vi "Give_Name_Cluster(Img_Setting)-1.vi"() -> (1 "Histogram Settings":T2, 2 "Image Settings":T1)   [LabVIEW 2013]
panel:
  in  "Expanding Factor":u16=700
  in  "Inverse #2":bool=TRUE
  in  "Inverse #1":bool=TRUE
  in  "Shift #2":u16
  in  "Shift #1":u16
  in  "Sigma #2":dbl=2.5
  in  "Dim #2":u8=15
  in  "Sigma #1":dbl=2.5
  in  "Dim #1":u8=15
  in  "Operator #2":T3(ring)
  in  "Intensity #2":sgl format="%.2f"
  in  "Operator #1":T3(ring)
  in  "Intensity #1":sgl format="%.2f"
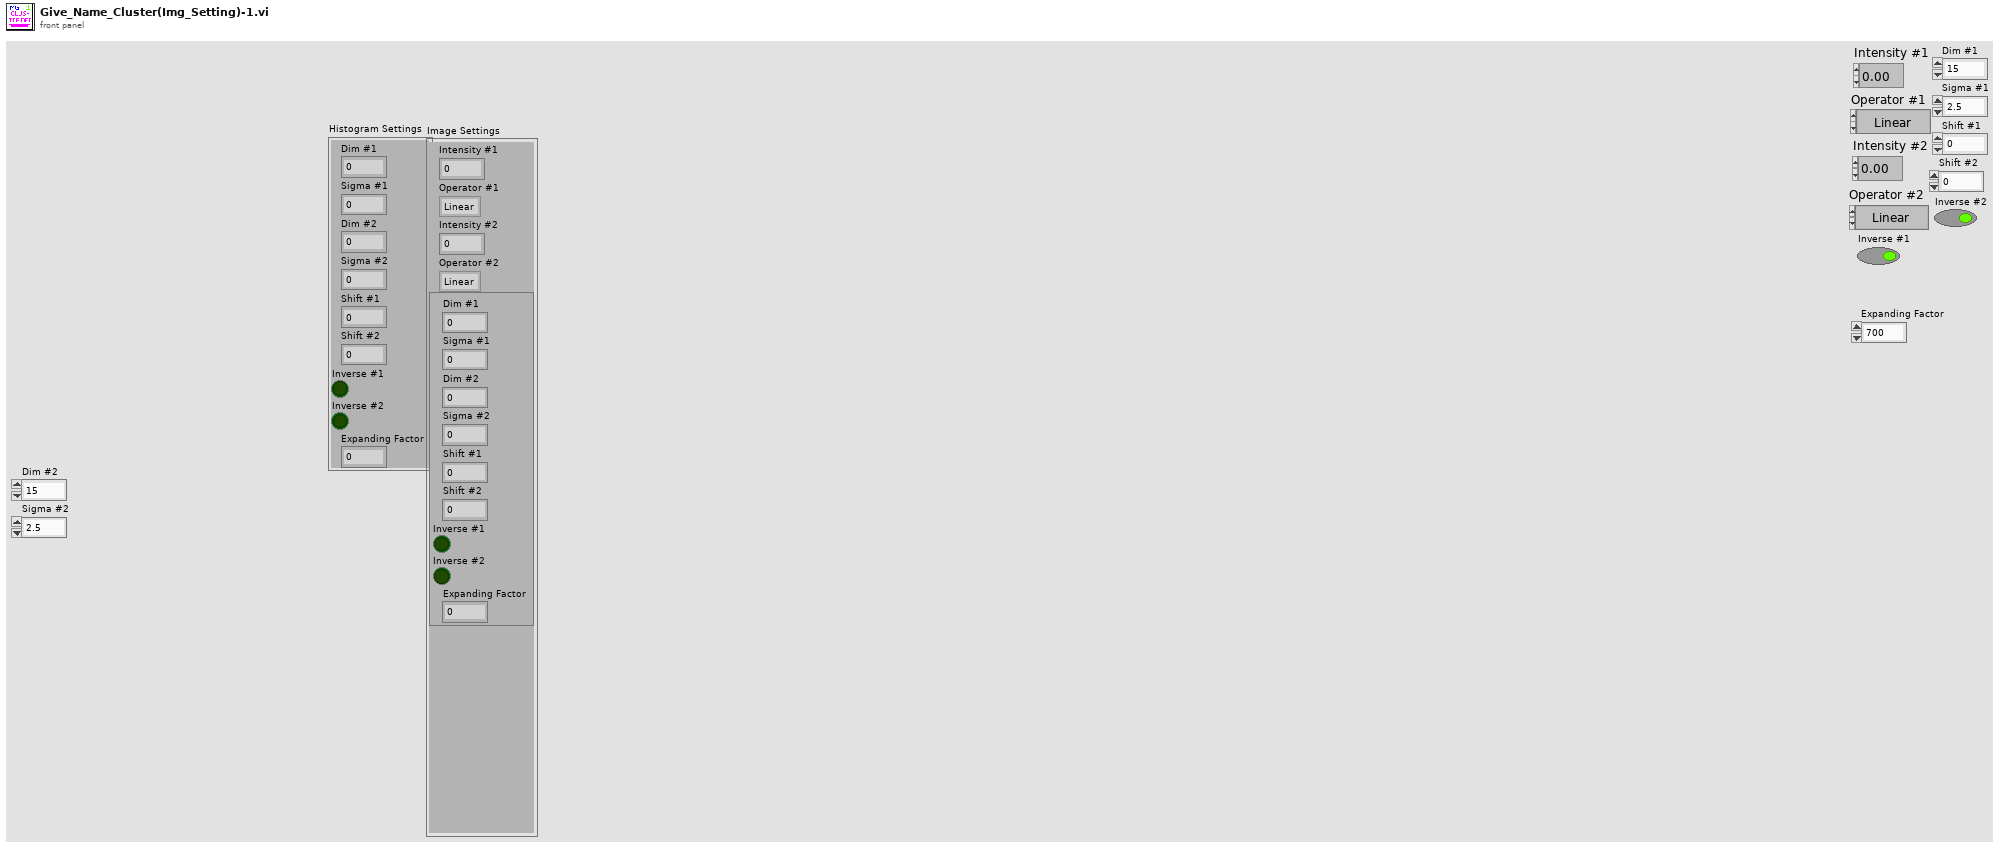
[diagram p1: front panel]
types:
  T1 = cluster{"Intensity #1":sgl, "Operator #1":enum32{"Linear", "Log", "Exp", "Square", "Square root", "Power X", "Power 1/X"}, "Intensity #2":sgl, "Operator #2":enum32{"Linear", "Log", "Exp", "Square", "Square root", "Power X", "Power 1/X"}, cluster{"Dim #1":u8, "Sigma #1":dbl, "Dim #2":u8, "Sigma #2":dbl, "Shift #1":u16, "Shift #2":u16, "Inverse #1":bool, "Inverse #2":bool, "Expanding Factor":u16}}
  T2 = cluster{"Dim #1":u8, "Sigma #1":dbl, "Dim #2":u8, "Sigma #2":dbl, "Shift #1":u16, "Shift #2":u16, "Inverse #1":bool, "Inverse #2":bool, "Expanding Factor":u16}
  T3 = enum32{"Linear", "Log", "Exp", "Square", "Square root", "Power X", "Power 1/X"}
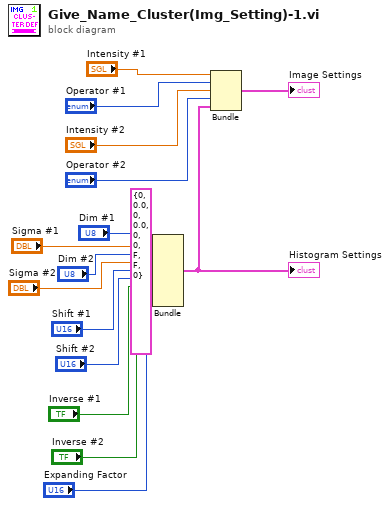
[diagram p0: block diagram]
diagram:
  (unwired) T2 {"Dim #1"=0, "Sigma #1"=0.0, "Dim #2"=0, "Sigma #2"=0.0, "Shift #1"=0, "Shift #2"=0, "Inverse #1"=FALSE, "Inverse #2"=FALSE, "Expanding Factor"=0} ("cluster")
  n1 = Bundle("Dim #1"="Dim #1", "Sigma #1"="Sigma #1", "Dim #2"="Dim #2", "Sigma #2"="Sigma #2", "Shift #1"="Shift #1", "Shift #2"="Shift #2", "Inverse #1"="Inverse #1", "Inverse #2"="Inverse #2", "Expanding Factor"="Expanding Factor") -> (w2:T2)  [unwired: 1 in]
  "Histogram Settings" <- w2
  n2 = Bundle("Intensity #1"="Intensity #1", "Operator #1"="Operator #1", "Intensity #2"="Intensity #2", "Operator #2"="Operator #2", w2) -> (→"Image Settings":T1)  [unwired: 1 in]
